vi "CCD spectrum processing_Shaowei-v2.vi"() -> ()   [LabVIEW 2009]
uses:
  <vilib>/Utility/file.llb/Read From Spreadsheet File (DBL).vi
panel:
  in  "select 2":bool
  in  "select":bool
  in  "next 2":bool
  in  "next":bool
  in  "previous 2":bool
  in  "previous":bool
  in  "?":bool
  out "?":path
  out "?":path
  out "?":string
  out "?":string
  in  "?":bool
  out "Spectrum 2":cluster{"Y":dbl[], "Y":dbl[]}[](graph)
  in  "?":bool=TRUE
  in  "?":bool
  out "Y":sgl
  out "X":sgl
  out "MIN":dbl
  out "MAX":dbl
  out "Spectrum 1":cluster{"Y":dbl[], "Y":dbl[]}[](graph)
  in  "?":bool
  in  "?":path=path "C:/Users/S. W. Li/Desktop/1.txt"
  in  "?":bool
  out "?":ext=1340.0
  in  "to":dbl=950.0
  in  "From":dbl=550.0
  in  "?":bool
  in  "?":i32(ring)=1 items=["nm"=1, "eV"=2, "cm-1"=3, "Pixel #"=4]
  # "Input File"
  # "2 Files"
  # "1 File"
  # "1st"
  # "2nd"
  # "Active Window"
  # "#1"
  # "#2"
  # "Spectra Range"
  # "nm"
  # "nm"
  # "# of Pixel"
  # "X unit"
  # "Cosmic Ray Removal"
  # "NO"
  # "YES"
  # "Value"
  # "Position"
  # "Save File"
  # "NO"
  # "YES"
  # "Descending"
  # "Sort Data by X"
  # "File Name"
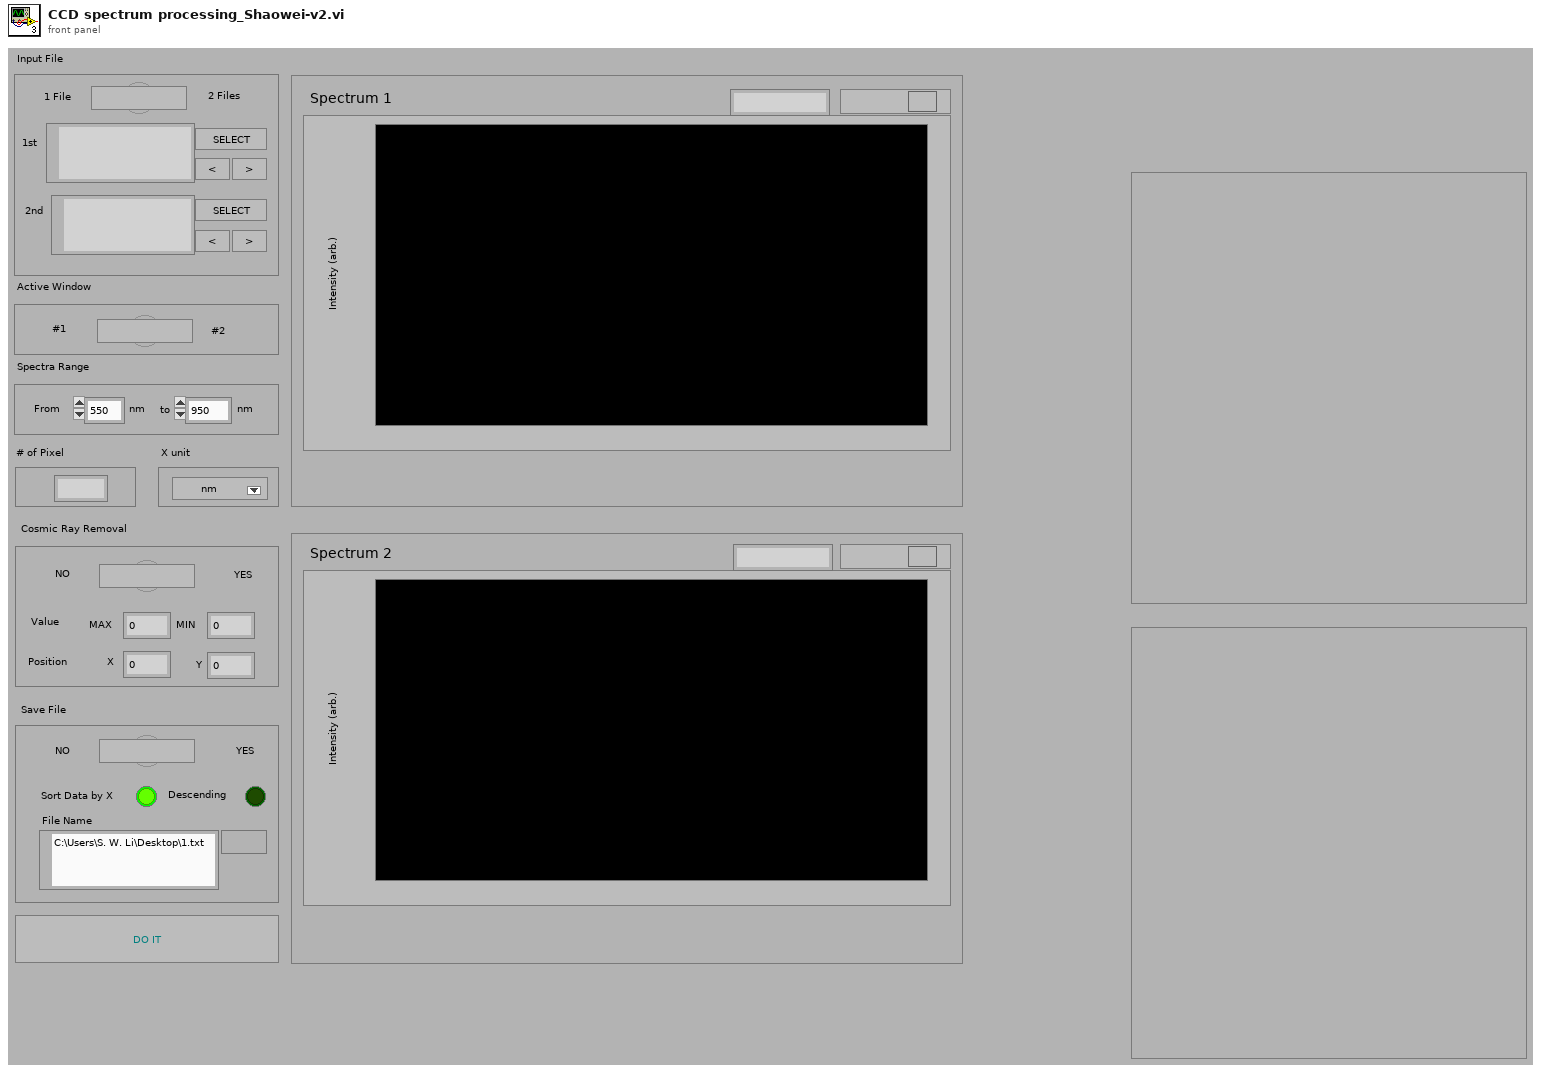
[diagram p1: front panel]
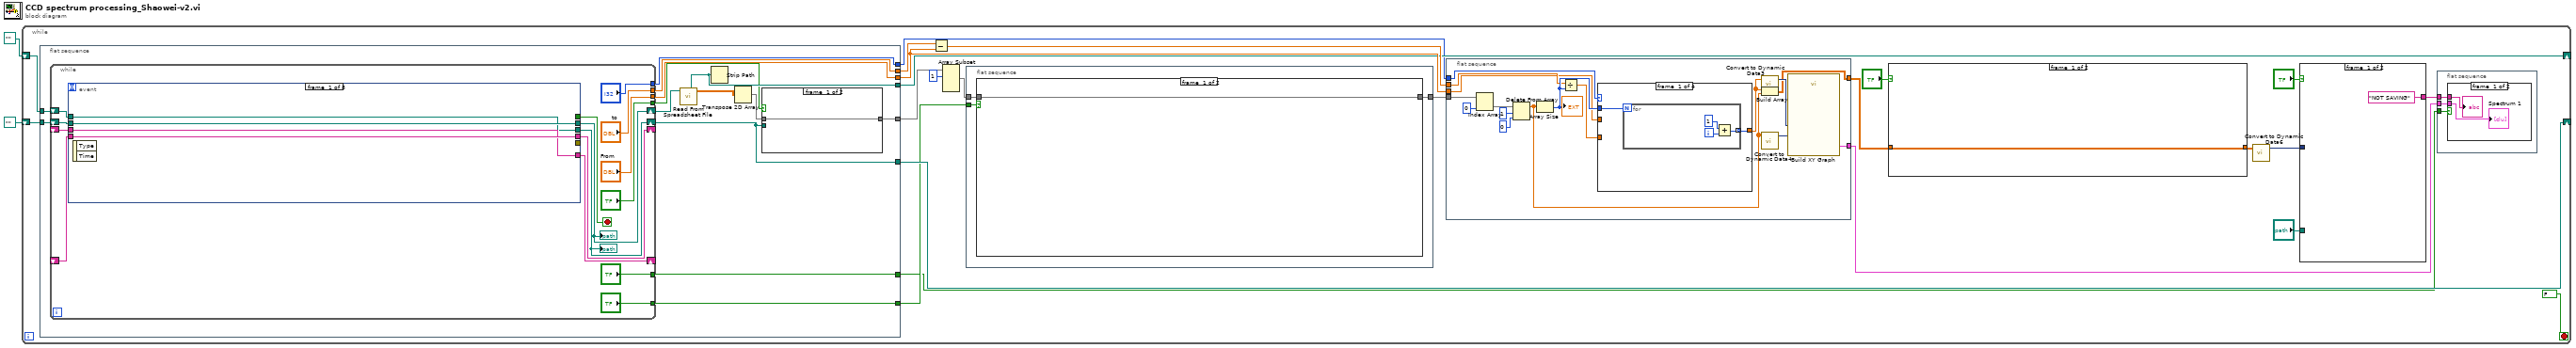
[diagram p0: block diagram]
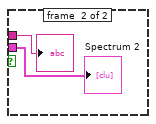
[diagram p2: hidden frame]
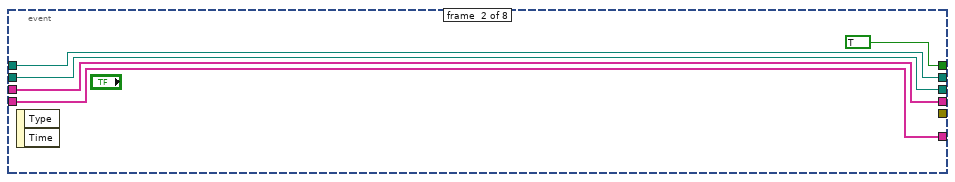
[diagram p3: hidden frame]
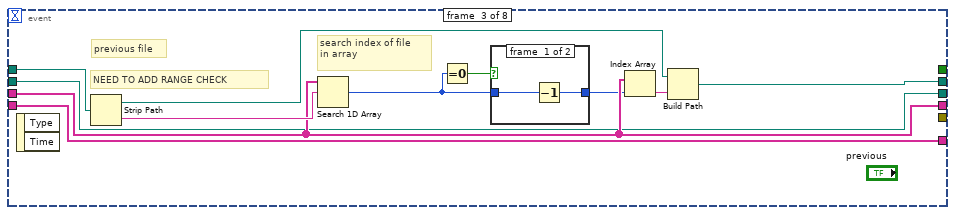
[diagram p4: hidden frame]
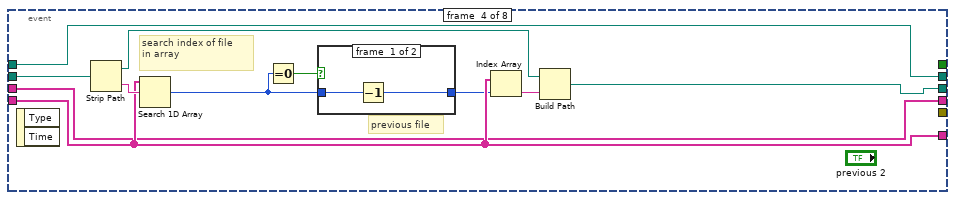
[diagram p6: hidden frame]
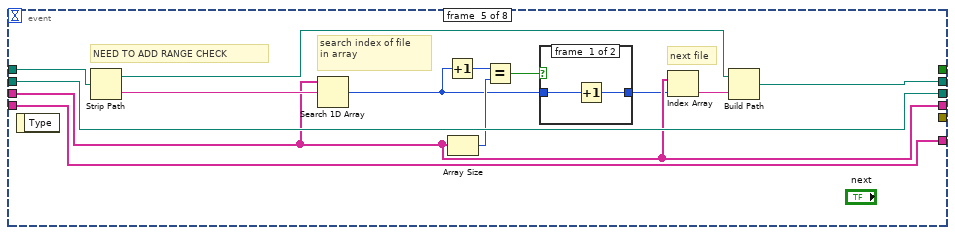
[diagram p8: hidden frame]
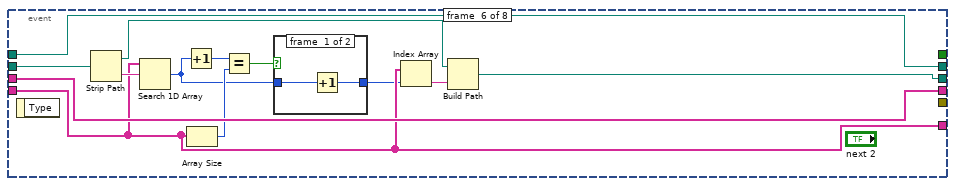
[diagram p10: hidden frame]
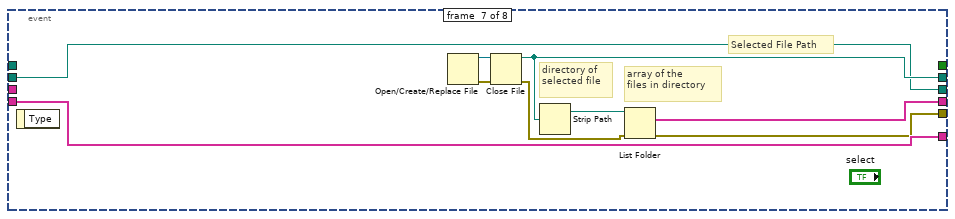
[diagram p12: hidden frame]
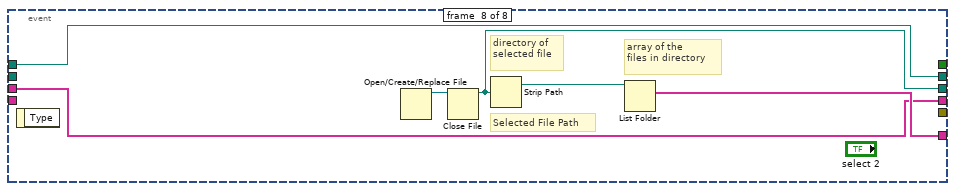
[diagram p13: hidden frame]
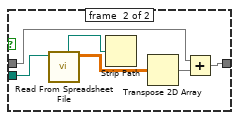
[diagram p14: hidden frame]
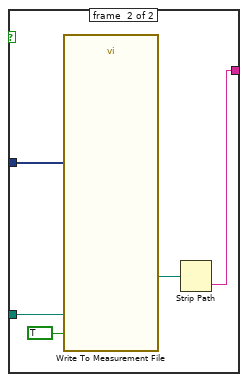
[diagram p15: hidden frame]
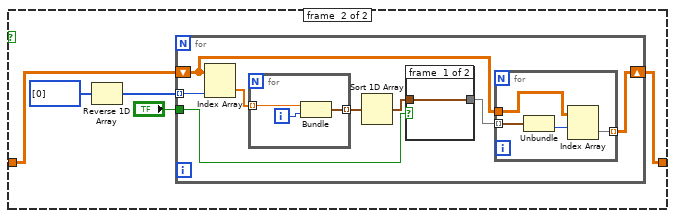
[diagram p16: hidden frame]
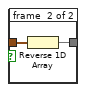
[diagram p17: hidden frame]
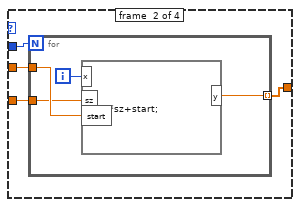
[diagram p18: hidden frame]
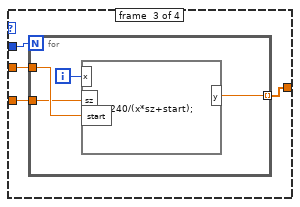
[diagram p19: hidden frame]
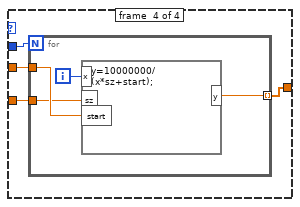
[diagram p20: hidden frame]
diagram:
  n1 = while {
    shift-right: [w7] -> _
    shift-left: path "" ("path") -> [w9]
    shift-right: [w6] -> _
    shift-left: path "" ("path") -> [w8]
    stop <- FALSE ("stop 2") stop-if-true
    n2 = flat-sequence {
      tunnel: [w44] -> w22
      tunnel: [w36] -> w11
      tunnel: [w35] -> w10
      tunnel: w9 -> [w42]
      tunnel: w8 -> [w41]
      tunnel: [w40] -> w7
      tunnel: [w39] -> w6
      tunnel: [w37] -> w5
      tunnel: [w34] -> w4
      tunnel: [w33] -> w3
      frame #0 {
        n3 = while {
          shift-right: [w60] -> _
          shift-left: _ -> [w59]
          shift-right: [w61] -> w43
          shift-left: w42 -> [w58]
          shift-right: [w57] -> w39
          shift-left: w41 -> [w56]
          shift-right: [w55] -> _
          shift-left: _ -> [w54]
          tunnel: ["?"] -> w38
          tunnel: ["?"] -> w37
          tunnel: ["to"] -> w36
          tunnel: ["From"] -> w35
          tunnel: ["?"] -> w34
          tunnel: ["?"] -> w33
          stop <- w53 stop-if-true
          n4 = event shown="[3] \"previous 2\": Value Change" {
            selector: _ -> [_ _ _ _ _ _ _ _]
            dyn-events: _ -> [_ _ _ _ _ _ _ _]
            timeout: _ -> [_ _ _ _ _ _ _ _]
            tunnel: [_ TRUE _ _ _ _ _ _] -> w53
            tunnel: [w64 w68 w76 w85 w108 w116 w136 w141] -> w61
            tunnel: [w65 w69 w78 w90 w101 w124 w137 w140] -> w60
            tunnel: w59 -> [w65 w69 w78 w90 w101 w124 _ w140]
            tunnel: w58 -> [w64 w68 w81 w85 w107 w116 _ w141]
            tunnel: [w62 w66 w74 w86 w105 w117 w134 w143] -> w57
            tunnel: w56 -> [w62 w66 w74 w92 w105 w115 w134 _]
            tunnel: [w63 w67 w75 w91 w106 w120 w135 w142] -> w55
            tunnel: w54 -> [w63 w67 w75 w91 w106 w120 w135 _]
            tunnel: [_ _ _ _ _ _ w131 _] -> _
            event #0 {
              n5 = event-data() -> ()  [unwired: 1 in, 2 out]
            }
            event #1 {
              n6 = event-data() -> ()  [unwired: 1 in, 2 out]
            }
            event #2 {
              # "NEED TO ADD RANGE CHECK"
              # "previous file"
              # "search index of file\nin array"
              n7 = event-data() -> ()  [unwired: 1 in, 2 out]
              n8 = Strip Path(path=w81) -> (stripped path=w79:path, name=w80:string)
              n9 = Search 1D Array(1D array=w78, element=w80) -> (index of element=w72:i32)  [unwired: 1 in]
              n10 = Equal To 0?(x=w72) -> (x = 0?=w73:bool)
              n11 = case shown="False" w73 {
                tunnel: w72 -> [w83 w84]
                tunnel: [w82 w84] -> w71
                frame #0 {
                  n12 = Decrement(x=w83) -> (x-1=w82:i32)
                }
                frame #1 {
                }
              }
              n13 = Index Array(array=w78, index=w71) -> (element=w77:string)
              n14 = Build Path(base path=w79, name or relative path=w77) -> (appended path=w76:path)
            }
            event #3 {
              # "previous file"
              # "search index of file\nin array"
              n15 = event-data() -> ()  [unwired: 1 in, 2 out]
              n16 = Strip Path(path=w92) -> (stripped path=w94:path, name=w95:string)
              n17 = Search 1D Array(1D array=w91, element=w95) -> (index of element=w88:i32)  [unwired: 1 in]
              n18 = Equal To 0?(x=w88) -> (x = 0?=w89:bool)
              n19 = case shown="False" w89 {
                tunnel: w88 -> [w97 w98]
                tunnel: [w96 w98] -> w87
                frame #0 {
                  n20 = Decrement(x=w97) -> (x-1=w96:i32)
                }
                frame #1 {
                }
              }
              n21 = Index Array(array=w91, index=w87) -> (element=w93:string)
              n22 = Build Path(base path=w94, name or relative path=w93) -> (appended path=w86:path)
            }
            event #4 {
              # "NEED TO ADD RANGE CHECK"
              # "next file"
              # "search index of file\nin array"
              n23 = event-data() -> ()  [unwired: 1 in, 1 out]
              n24 = Strip Path(path=w107) -> (stripped path=w110:path, name=w111:string)
              n25 = Search 1D Array(1D array=w101, element=w111) -> (index of element=w100:i32)  [unwired: 1 in]
              n26 = Increment(x=w100) -> (x+1=w102:i32)
              n27 = Array Size(array=w101) -> (size(s)=w104:i32)
              n28 = Equal?(x=w102, y=w104) -> (x = y?=w103:bool)
              n29 = case shown="True" w103 {
                tunnel: w100 -> [w113 w114]
                tunnel: [w112 w114] -> w99
                frame #0 {
                  n30 = Increment(x=w113) -> (x+1=w112:i32)
                }
                frame #1 {
                }
              }
              n31 = Index Array(array=w101, index=w99) -> (element=w109:string)
              n32 = Build Path(base path=w110, name or relative path=w109) -> (appended path=w108:path)
            }
            event #5 {
              n33 = event-data() -> ()  [unwired: 1 in, 1 out]
              n34 = Strip Path(path=w115) -> (stripped path=w126:path, name=w127:string)
              n35 = Search 1D Array(1D array=w120, element=w127) -> (index of element=w119:i32)  [unwired: 1 in]
              n36 = Increment(x=w119) -> (x+1=w121:i32)
              n37 = Array Size(array=w120) -> (size(s)=w123:i32)
              n38 = Equal?(x=w121, y=w123) -> (x = y?=w122:bool)
              n39 = case shown="True" w122 {
                tunnel: w119 -> [w129 w130]
                tunnel: [w128 w130] -> w118
                frame #0 {
                  n40 = Increment(x=w129) -> (x+1=w128:i32)
                }
                frame #1 {
                }
              }
              n41 = Index Array(array=w120, index=w118) -> (element=w125:string)
              n42 = Build Path(base path=w126, name or relative path=w125) -> (appended path=w117:path)
            }
            event #6 {
              # "array of the \nfiles in directory"
              # "directory of\nselected file"
              # "Selected File Path"
              n43 = event-data() -> ()  [unwired: 1 in, 1 out]
              n44 = Open/Create/Replace File() -> (refnum out=w139:refnum<file>, error out=w133:errorcluster)  [unwired: 6 in, 1 out]
              n45 = Close File(refnum=w139, error in=w133) -> (path=w136:path, error out=w132:errorcluster)
              n46 = Strip Path(path=w136) -> (stripped path=w138:path)  [unwired: 1 out]
              n47 = List Folder(path=w138, error in=w132) -> (filenames=w137:string[], error out=w131:errorcluster)  [unwired: 2 in, 2 out]
            }
            event #7 {
              # "array of the \nfiles in directory"
              # "directory of\nselected file"
              # "Selected File Path"
              n48 = event-data() -> ()  [unwired: 1 in, 1 out]
              n49 = Open/Create/Replace File() -> (refnum out=w145:refnum<file>)  [unwired: 6 in, 2 out]
              n50 = Close File(refnum=w145) -> (path=w143:path)  [unwired: 1 in, 1 out]
              n51 = Strip Path(path=w143) -> (stripped path=w144:path)  [unwired: 1 out]
              n52 = List Folder(path=w144) -> (filenames=w142:string[])  [unwired: 3 in, 3 out]
            }
          }
          "?" <- w61
          "?" <- w57
        }
        n53 = call-poly <vilib>:"Read From Spreadsheet File.vi"("file path (dialog if empty)"=w43) -> ("all rows"=w46:dbl[][], "new file path (Not A Path if cancelled)"=w40:path)  [unwired: 6 in, 3 out]
        n54 = Strip Path(path=w40) -> ()  [unwired: 2 out]
        n55 = Transpose 2D Array(2D array=w46) -> (transposed array=w45:dbl[][])
        n56 = case shown="False" w38 {
          tunnel: w45 -> [w146 w151]
          tunnel: [w146 w150] -> w44
          tunnel: w39 -> [_ w147]
          frame #0 {
          }
          frame #1 {
            n57 = call-poly <vilib>:"Read From Spreadsheet File.vi"("file path (dialog if empty)"=w147) -> ("all rows"=w149:dbl[][], "new file path (Not A Path if cancelled)"=w152:path)  [unwired: 6 in, 3 out]
            n58 = Strip Path(path=w152) -> ()  [unwired: 2 out]
            n59 = Transpose 2D Array(2D array=w149) -> (transposed array=w148:dbl[][])
            n60 = Add(x=w151, y=w148) -> (x+y=w150:dbl[][])
          }
        }
      }
    }
    n61 = Subtract(x=w11, y=w10) -> (x-y=w20:dbl)
    n62 = Array Subset(array=w22, index (row)=1) -> (w25:dbl[][])  [unwired: 3 in]
    n63 = flat-sequence {
      tunnel: w25 -> [w230]
      tunnel: w5 -> [w229]
      tunnel: [w228] -> w21
      frame #0 {
        n64 = case shown="False" w229 {
          tunnel: w230 -> [w231 w235]
          tunnel: [w231 w233] -> w228
          frame #0 {
          }
          frame #1 {
            n65 = Transpose 2D Array(2D array=w235) -> (transposed array=w234:dbl[][])
            n66 = while {
              shift-right: [w272] -> w232
              shift-left: w234 -> [w236]
              stop <- w251 stop-if-true
              w249 = 3
              n67 = Array Max & Min(array=w236) -> (max value=→"MAX":dbl, max index (indices)=w270:i32[], min value=→"MIN":dbl)  [unwired: 1 out]
              n68 = local read "Y"() -> (w238:sgl)
              n69 = Subtract(x=w238, y=5) -> (x-y=w266:sgl)
              n70 = Index Array(array=w270, index=0) -> (element=w243:i32)
              "X" <- w243
              n71 = Index Array(array=w270, index=1) -> (element=w242:i32)
              "Y" <- w242
              n72 = local read "X"() -> (w239:sgl)
              n73 = Array Subset(array=w236, index (row)=w239, length (row)=1, index (col)=w266, length (col)=w249) -> (w248:dbl[][])
              n74 = Subtract(x=w238, y=1) -> (x-y=w265:sgl)
              n75 = Add Array Elements(numeric array=w248) -> (sum=w250:dbl)
              n76 = Replace Array Subset(array=w236, new element=w248, index (row)=w239, index (col)=w265) -> (w272:dbl[][])
              n77 = Subtract(x=w238, y=2) -> (x-y=w261:sgl)
              n78 = Subtract(x=w242, y=2) -> (x-y=w256:i32)
              n79 = Divide(x=w250, y=w249) -> (x/y=w247:dbl)
              n80 = Array Subset(array=w236, index (row)=w243, length (row)=1, index (col)=w256, length (col)=5) -> (w254:dbl[][])
              n81 = Array Subset(array=w272, index (row)=w239, length (row)=1, index (col)=w261, length (col)=5) -> (w259:dbl[][])
              n82 = Multiply(x=w247, y=1.2) -> (x*y=w252:dbl)
              n83 = local read "MAX"() -> (w237:dbl)
              n84 = call "Convert to Dynamic Data"("2D Array"=w254) -> ("Dynamic Data Type"=w246:dynamicdata)  [unwired: 3 in]
              n85 = call "Convert to Dynamic Data2"("2D Array"=w259) -> ("Dynamic Data Type"=w244:dynamicdata)  [unwired: 3 in]
              n86 = Less?(x=w237, y=w252) -> (x < y?=w251:bool)
              n87 = Merge Signals(w246, w244) -> (w245:dynamicdata)
              n88 = call "Build Table"("Signals"=w245) -> ()  [unwired: 9 in, 2 out]
            }
            n89 = Transpose 2D Array(2D array=w232) -> (transposed array=w233:dbl[][])
          }
        }
      }
    }
    n90 = flat-sequence {
      tunnel: w21 -> [w198]
      tunnel: [w190] -> w19
      tunnel: w4 -> [w188]
      tunnel: w20 -> [w186]
      tunnel: w10 -> [w185]
      tunnel: [w183] -> w15
      frame #0 {
        n91 = Index Array(array=w198, index (col)=0) -> (element=w193:dbl[])  [unwired: 1 in]
        n92 = Delete From Array(array=w193, length=1, index=0) -> (array with subset deleted=w192:dbl[])  [unwired: 1 out]
        n93 = Array Size(array=w192) -> (size(s)=w187:i32)
        "?" <- w187
        n94 = Divide(x=w186, y=w187) -> (x/y=w184:dbl)
        n95 = case shown="4, Default" w188 {
          tunnel: w187 -> [w200 w207 w215 w223]
          tunnel: [w199 w206 w214 w222] -> w191
          tunnel: w185 -> [_ w205 w213 w221]
          tunnel: w184 -> [_ w204 w212 w220]
          frame #0 {
            n96 = for {
              N: w200 -> [_]
              tunnel: [w201] -> w199 mode=indexing
              i -> [w202]
              n97 = Add(x=1, y=w202) -> (x+y=w201:i32)
            }
          }
          frame #1 {
            n98 = for {
              N: w207 -> [_]
              tunnel: [w208] -> w206 mode=indexing
              tunnel: w205 -> [w210]
              tunnel: w204 -> [w209]
              i -> [w211]
              n99 = formula code="y=x*sz+start;"("x"=w211, "sz"=w209, "start"=w210) -> ("y"=w208:dbl)
            }
          }
          frame #2 {
            n100 = for {
              N: w215 -> [_]
              tunnel: [w216] -> w214 mode=indexing
              tunnel: w213 -> [w218]
              tunnel: w212 -> [w217]
              i -> [w219]
              n101 = formula code="y=1240/(x*sz+start);"("x"=w219, "sz"=w217, "start"=w218) -> ("y"=w216:dbl)
            }
          }
          frame #3 {
            n102 = for {
              N: w223 -> [_]
              tunnel: [w224] -> w222 mode=indexing
              tunnel: w221 -> [w226]
              tunnel: w220 -> [w225]
              i -> [w227]
              n103 = formula code="y=10000000/(x*sz+start);"("x"=w227, "sz"=w225, "start"=w226) -> ("y"=w224:dbl)
            }
          }
        }
        n104 = call "Convert to Dynamic Data3"("Array"=w191) -> ("Dynamic Data Type"=w197:dynamicdata)  [unwired: 3 in]
        n105 = Build Array(w191, w192) -> (w190:dbl[][])
        n106 = call "Convert to Dynamic Data4"("Array"=w192) -> ("Dynamic Data Type"=w196:dynamicdata)  [unwired: 3 in]
        n107 = call "Build XY Graph"("Y Input"=w196, "X Input"=w197) -> ("XY Graph"=w183:cluster{"Y":dbl[], "Y":dbl[]}[])  [unwired: 8 in, 1 out]
      }
    }
    n108 = case shown="True" "?" {
      tunnel: w19 -> [w159 w161]
      tunnel: [w159 w160] -> w16
      frame #0 {
      }
      frame #1 {
        n109 = Reverse 1D Array(array=i32[] [0] ("Priority Columns (0)")) -> (reversed array=w163:i32[])
        n110 = for {
          shift-right: [w166] -> w160
          shift-left: w161 -> [w168]
          tunnel: w163 -> [w165] mode=indexing
          tunnel: "?" -> [w167]
          n111 = Index Array(array=w168, index (col)=w165) -> (element=w170:dbl[])  [unwired: 1 in]
          n112 = for {
            tunnel: w170 -> [w180] mode=indexing
            tunnel: [w182] -> w169 mode=indexing
            i -> [w181]
            n113 = Bundle("y"=w180, w181) -> (w182:cluster{"y":dbl, i32})  [unwired: 1 out]
          }
          n114 = Sort 1D Array(array=w169) -> (sorted array=w172:cluster{"y":dbl, i32}[])
          n115 = case shown="True" w167 {
            tunnel: [w173 w174] -> w171
            tunnel: w172 -> [w173 w175]
            frame #0 {
            }
            frame #1 {
              n116 = Reverse 1D Array(array=w175) -> (reversed array=w174:cluster{"y":dbl, i32}[])
            }
          }
          n117 = for {
            tunnel: w171 -> [w179] mode=indexing
            tunnel: w168 -> [w178]
            tunnel: [w176] -> w166 mode=indexing
            n118 = Unbundle(w179) -> (w177:i32)  [unwired: 1 out]
            n119 = Index Array(array=w178, index (row)=w177) -> (element=w176:dbl[])  [unwired: 1 in]
          }
        }
      }
    }
    n120 = call "Convert to Dynamic Data6"("2D Array"=w16) -> ("Dynamic Data Type"=w18:dynamicdata)  [unwired: 3 in]
    n121 = case shown="True" "?" {
      tunnel: w18 -> [_ w158]
      tunnel: "?" -> [_ w157]
      tunnel: ["NOT SAVING" ("name") w154] -> w12
      frame #0 {
      }
      frame #1 {
        n122 = call "Write To Measurement File"("Signals"=w158, "Reset"=TRUE, "Filename"=w157) -> ("Filename Out"=w155:path)  [unwired: 14 in, 2 out]
        n123 = Strip Path(path=w155) -> (name=w154:string)  [unwired: 1 out]
      }
    }
    n124 = flat-sequence {
      tunnel: w15 -> [w28]
      tunnel: w12 -> [w27]
      tunnel: w3 -> [w26]
      frame #0 {
        n125 = case shown="False" w26 {
          tunnel: w28 -> [w30 w32]
          tunnel: w27 -> [w29 w31]
          frame #0 {
            "Spectrum 1" <- w30
            "?" <- w29
          }
          frame #1 {
            "Spectrum 2" <- w32
            "?" <- w31
          }
        }
      }
    }
  }
